vi "Set Ring Strings and Values by String and Value array.vi"(8 "error in (no error)":errorcluster, 10 "Strings And Values []":T1, 11 "Ring Field in":refnum<class "Ring Field.lvclass">) -> (0 "error out":errorcluster, 3 "Ring Field out":refnum<class "Ring Field.lvclass">)   [LabVIEW 2020, in "Ring Field.lvclass"]
uses:
  Ring Field.lvclass
  <vilib>/Utility/miscctls.llb/LVStringsAndValuesArrayTypeDef.ctl
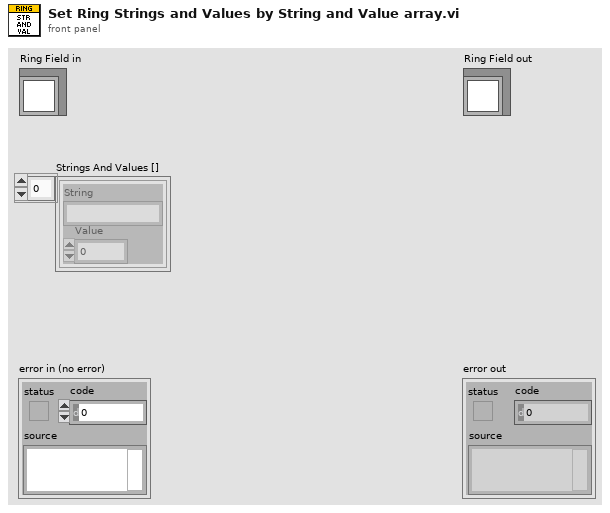
[diagram p1: front panel]
types:
  T1 = typedef "LVStringsAndValuesArrayTypeDef.ctl" = cluster{"String":string, "Value":ext}[]
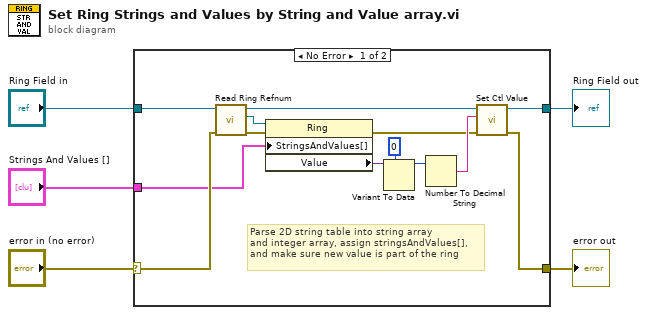
[diagram p0: block diagram]
diagram:
  n1 = case shown="No Error" "error in (no error)" {
    selector: "error in (no error)" -> [w8 w20]
    tunnel: [w7 w20] -> w4
    tunnel: [w11 w19] -> w2
    tunnel: "Ring Field in" -> [w18 w19]
    tunnel: "Strings And Values []" -> [w6 _]
    frame No Error {
      # "Parse 2D string table into string array\nand integer array, assign stringsAndValues[],\nand make sure new value is part of the ring"
      n2 = call "Read Ring Refnum.vi"("error in (no error)"=w8, "Ring Field in"=w18) -> ("error out"=w16:errorcluster, "Ring Refnum"=w17:refnum<vi>, "Ring Field out"=w12:refnum<class "Ring Field.lvclass">)  [unwired: 7 in]
      n3 = property class="Ring"(reference=w17, error in=w16, "StringsAndValues[]"=w6) -> (error out=w9:errorcluster, "Value"=w15:variant)  [unwired: 1 out]
      n4 = Variant To Data(type=0, Variant=w15) -> (data=w13:i32)  [unwired: 1 in, 1 out]
      n5 = Number To Decimal String(number=w13) -> (decimal integer string=w10:string)  [unwired: 1 in]
      n6 = call-dynamic "Set Ctl Value.vi"("error in (no error)"=w9, "String"=w10, "Ring Field in"=w12) -> ("error out"=w7:errorcluster, "Ring Field out"=w11:refnum<class "Ring Field.lvclass">)  [unwired: 7 in]
    }
    frame Error {
    }
  }
  "error out" <- w4
  "Ring Field out" <- w2
